vi "test-single-jointed-arm-sim.vi"(8 "error in (no error)":errorcluster) -> (0 "error out":errorcluster, 3 "Test Passed":bool)   [LabVIEW 2019]
uses:
  <vilib>/Rock Robotics/WPI/ThirdParty/JAS_Junk/TrajLib/DCMOTOR.CTL
  <vilib>/Rock Robotics/WPI/ThirdParty/JAS_Junk/TrajLib/SINGLE_JOINT_ARM_SIM.ctl
  <vilib>/Rock Robotics/WPI/ThirdParty/JAS_Junk/TrajLib/LINEAR_SYSTEM_SIM.ctl
  <vilib>/Rock Robotics/WPI/ThirdParty/JAS_Junk/TrajLib/LINEAR_SYSTEM.ctl
  <vilib>/Analysis/Matrix/Datatypes/RealMatrix.ctl
  <vilib>/Rock Robotics/WPI/ThirdParty/JAS_Junk/TrajLib/MatBuilder_Create.vi
  <vilib>/Rock Robotics/WPI/ThirdParty/JAS_Junk/TrajLib/DCMotor_New.vi
  <vilib>/Rock Robotics/WPI/ThirdParty/JAS_Junk/TrajLib/Units_RotationsPerMinuteToRadiansPerSecond.vi
  <vilib>/Rock Robotics/WPI/ThirdParty/JAS_Junk/TrajLib/Trajectory_Library.lvlib
  <vilib>/Analysis/Matrix/NI_Matrix.lvlib
panel:
  in  "Tab Control":enum32{"Operation", "Motor", "Arm Sim"}(tab)
  out "Velocity RAD/SEC":cluster{"Voltage":dbl}(graph)
  out "PV Chart":cluster{dbl}(graph)
  out "Position RAD":dbl
  in  "Input_Voltage":dbl format="%#_13g"
  out "Arm Motor":T1 {"Jr_KgM2" format="%13.5p"; "L_H" format="%13.5p"; "Kt_NMPerAmp" format="%13.5p"; "KvINV_RadPerSecPerVolt" format="%13.5p"; "R_Ohms" format="%13.5p"; "FreeSpeed_RadPerSec" format="%13.5p"; "FreeCurrent_Amps" format="%13.5p"; "StallCurrent_Amps" format="%13.5p"; "StallTorque_NM" format="%13.5p"; "nominalVoltage_Volts" format="%13.5p"}
  out "Arm Simulaation":T2 {"GearBox"."Jr_KgM2" format="%13.5p"; "GearBox"."L_H" format="%13.5p"; "GearBox"."Kt_NMPerAmp" format="%13.5p"; "GearBox"."KvINV_RadPerSecPerVolt" format="%13.5p"; "GearBox"."R_Ohms" format="%13.5p"; "GearBox"."FreeSpeed_RadPerSec" format="%13.5p"; "GearBox"."FreeCurrent_Amps" format="%13.5p"; "GearBox"."StallCurrent_Amps" format="%13.5p"; "GearBox"."StallTorque_NM" format="%13.5p"; "GearBox"."nominalVoltage_Volts" format="%13.5p"}
  # "<States, 1>"
  # "<Outputs, 1>"
  # "<Inputs, 1>"
  # "<Outputs, 1>"
  # "<States,States>"
  # "<States,Inputs>"
  # "<Outputs,States>"
  # "<Outputs,Inputs>"
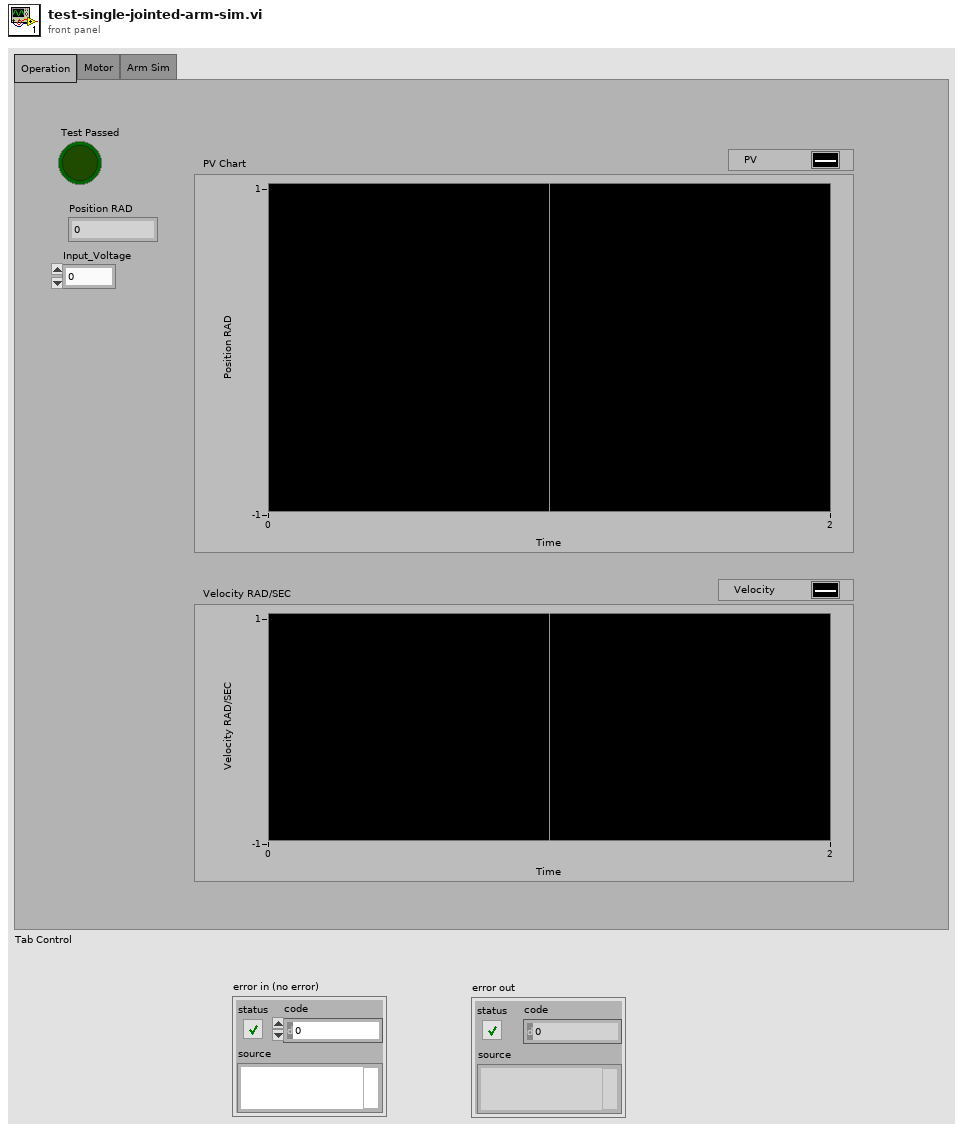
[diagram p1: front panel]
types:
  T1 = typedef "Trajectory_Library.lvlib/DCMOTOR.CTL" = cluster{"nominalVoltage_Volts":dbl, "StallTorque_NM":dbl, "StallCurrent_Amps":dbl, "FreeCurrent_Amps":dbl, "FreeSpeed_RadPerSec":dbl, "R_Ohms":dbl, "KvINV_RadPerSecPerVolt":dbl, "Kt_NMPerAmp":dbl, "L_H":dbl, "Jr_KgM2":dbl}
  T2 = typedef "Trajectory_Library.lvlib/SINGLE_JOINT_ARM_SIM.ctl" = cluster{"Arm_LinearSystem":T3, "GearBox":T1, "Gearing":dbl, "R_ArmLength_M":dbl, "MinAngle_Rad":dbl, "MaxAngle_Rad":dbl, "ArmMass_Kg":dbl, "SimulateGravity":bool}
  T3 = typedef "Trajectory_Library.lvlib/LINEAR_SYSTEM_SIM.ctl" = cluster{"m_Plant":T4, "m_X":T5, "m_Y":T5, "m_U":T5, "MeasureStdDev":T5}
  T4 = typedef "Trajectory_Library.lvlib/LINEAR_SYSTEM.ctl" = cluster{"m_A":T5, "m_B":T5, "m_C":T5, "m_D":T5, "States":i32, "Inputs":i32, "Outputs":i32}
  T5 = typedef "NI_Matrix.lvlib/RealMatrix.ctl" = dbl[][]
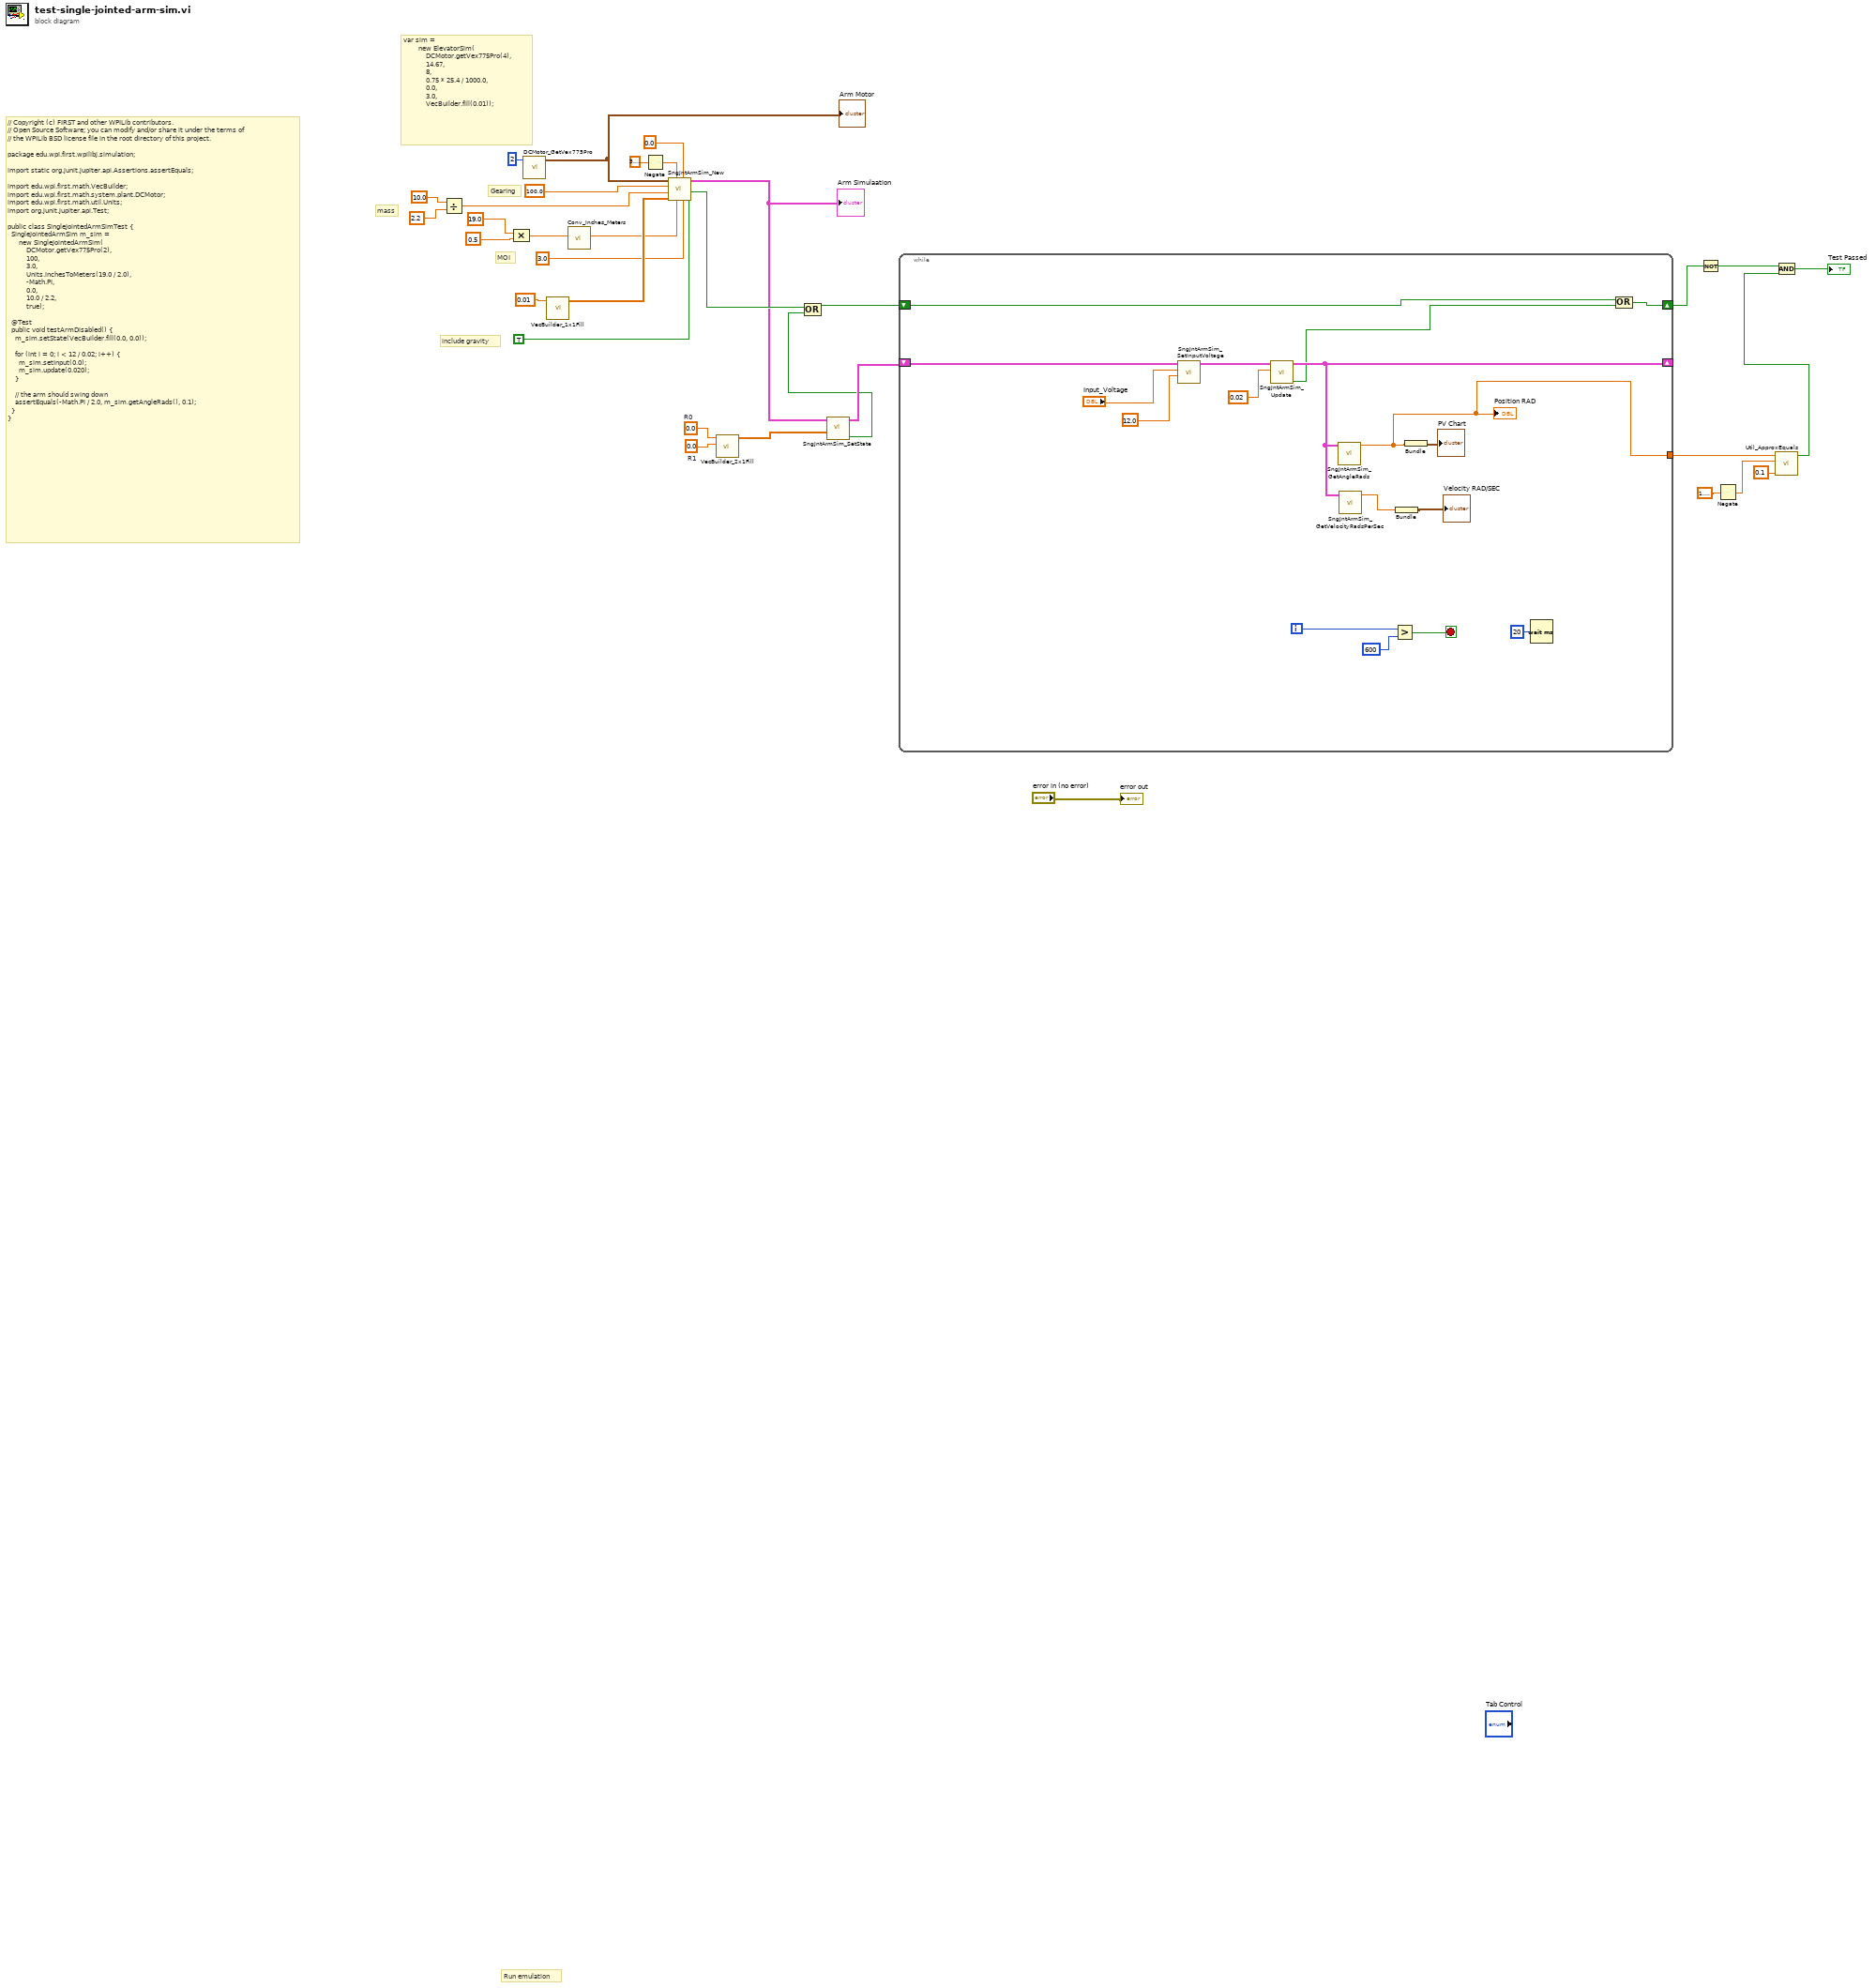
[diagram p0: block diagram]
diagram:
  w6 = 0.0  # R1
  w5 = 0.0  # R0
  # "include gravity"
  # "MOI"
  # "Gearing"
  # "// Copyright (c) FIRST and other WPILib contributors.\n// Open Source Software; you can modify and/or share it under the terms of\n// the WPILib BSD license file in the root directory of this project.\n\npackage edu.wpi.first.wpilibj.simulation;\n\nimport static org.junit.jupiter.api.Assertions.assertEquals;\n\nimport edu.wpi.first.math.VecBuilder;\nimport edu.wpi.first.math.system.plant.DCMotor;\nimport edu.wpi.first.math.util.Units;\nimport org.junit.jupiter.api.Test;\n\npublic class SingleJointedArmSimTest {\n  SingleJointedArmSim m_sim =\n      new SingleJointedArmSim(\n          DCMotor.getVex775Pro(2),\n          100,\n          3.0,\n          Units.inchesToMeters(19.0 / 2.0),\n          -Math.PI,\n          0.0,\n          10.0 / 2.2,\n          true);\n\n  @Test\n  public void testArmDisabled() {\n    m_sim.setState(VecBuilder.fill(0.0, 0.0));\n\n    for (int i = 0; i < 12 / 0.02; i++) {\n      m_sim.setInput(0.0);\n      m_sim.update(0.020);\n    }\n\n    // the arm should swing down\n    assertEquals(-Math.PI / 2.0, m_sim.getAngleRads(), 0.1);\n  }\n}"
  # "var sim =\n        new ElevatorSim(\n            DCMotor.getVex775Pro(4),\n            14.67,\n            8,\n            0.75 * 25.4 / 1000.0,\n            0.0,\n            3.0,\n            VecBuilder.fill(0.01));"
  # "mass"
  # "Run emulation"
  n1 = Divide(x=10.0, y=2.2) -> (x/y=w11:dbl)
  n2 = Compound Arithmetic op=MULTIPLY(19.0 ("value"), 0.5 ("value")) -> (w18:dbl)
  n3 = call <vilib>:"DCMotor_GetVex775Pro.vi"("Num Motors"=2) -> ("DCMOTOR"=w28:T1)  [unwired: 10 in]
  "Arm Motor" <- w28
  n4 = call <vilib>:"VecBuilder_1x1Fill.vi"("R0_C0"=0.01) -> ("output matrix"=w26:T5)  [unwired: 10 in]
  n5 = call <vilib>:"Conv_Inches_Meters.vi"("INCH"=w18) -> ("Meters"=w17:dbl)  [unwired: 10 in]
  n6 = Negate(x=3.141592653589793) -> (-x=w15:dbl)
  n7 = call <vilib>:"SngJntArmSim_New.vi"("SimulateGravity"=TRUE, "jKgMetersSquared"=3.0, "MaxAngle_Rad"=0.0 ("MaxHeight_Meters"), "ArmLength_Meters"=w17, "MinAngle_Rad"=w15, "MeasurementStdDev"=w26, "ArmMass_Kg"=w11, "Gearing"=100.0, "GearBox"=w28) -> ("Error"=w25:bool, "SingleJointArmSim"=w9:T2)  [unwired: 1 in]
  "Arm Simulaation" <- w9
  n8 = call <vilib>:"VecBuilder_2x1Fill.vi"("R1"=w6, "R0"=w5) -> ("output matrix"=w4:T5)  [unwired: 9 in]
  n9 = call <vilib>:"SngJntArmSim_SetState.vi"("System State"=w4, "in ArmSim"=w9) -> ("Size Coerced"=w7:bool, "out ArmSim"=w8:T2)  [unwired: 8 in]
  n10 = Compound Arithmetic op=OR(w25, w7) -> (w32:bool)
  n11 = while {
    shift-right: [w38] -> _
    shift-left: w8 -> [w40]
    shift-right: [w47] -> w21
    shift-left: w32 -> [w48]
    tunnel: [w36] -> w10
    i -> [w51]
    stop <- w49 stop-if-true
    n12 = call <vilib>:"SngJntArmSim_SetInputVoltage.vi"("Battery_Volts"=12.0, "Input_Voltage"="Input_Voltage", "in SingleJointArmSim"=w40) -> ("out SingleJointArmSim"=w45:T2)  [unwired: 8 in]
    n13 = call <vilib>:"SngJntArmSim_Update.vi"("dT_Seconds"=0.02, "in SingleJointArmSim"=w45) -> ("Error"=w35:bool, "out SingleJointArmSim"=w38:T2)  [unwired: 8 in]
    n14 = call <vilib>:"SngJntArmSim_GetAngleRads.vi"("SingleJointArmSim"=w38) -> ("ArmAngle_Rad"=w36:dbl)  [unwired: 10 in]
    "Position RAD" <- w36
    n15 = call <vilib>:"SngJntArmSim_GetVelocityRadsPerSec.vi"("singleJointArmSim"=w38) -> ("Velocity_RadsPerSec"=w37:dbl)  [unwired: 10 in]
    n16 = Greater?(x=w51, y=600) -> (0:w49:bool)
    n17 = Bundle("Velocity_RadsPerSec"=w37) -> (→"Velocity RAD/SEC":cluster{"Velocity_RadsPerSec":dbl})  [unwired: 1 in]
    n18 = Bundle("ArmAngle_Rad"=w36) -> (→"PV Chart":cluster{"ArmAngle_Rad":dbl})  [unwired: 1 in]
    n19 = Wait (ms)(milliseconds to wait=u32 20) -> ()  [unwired: 1 out]
    n20 = Compound Arithmetic op=OR(w48, w35) -> (w47:bool)
  }
  n21 = Not(x=w21) -> (.not. x?=w20:bool)
  n22 = Negate(x=1.5707963267948966) -> (-x=w2:dbl)
  n23 = call <vilib>:"Util_ApproxEquals.vi"("Tolerance"=0.1, "Value 2"=w2, "Value 1"=w10) -> ("ApproxEquals"=w22:bool)  [unwired: 8 in]
  n24 = Compound Arithmetic op=AND(w20, w22) -> (→"Test Passed":bool)
  "error out" <- "error in (no error)"
